vi "Module Info.vi"(8 "error in (no error)":errorcluster, 11 "BoardHandle":T2) -> (0 "error out":errorcluster, 2 "Module Info":T1, 3 "BoardHandle out":T2)   [LabVIEW 2020, in "CAEN PSM.lvlib"]
doc: "This function returns some information of the board."
uses:
  CAEN PSM.lvlib
  Private/BoardHandle.ctl
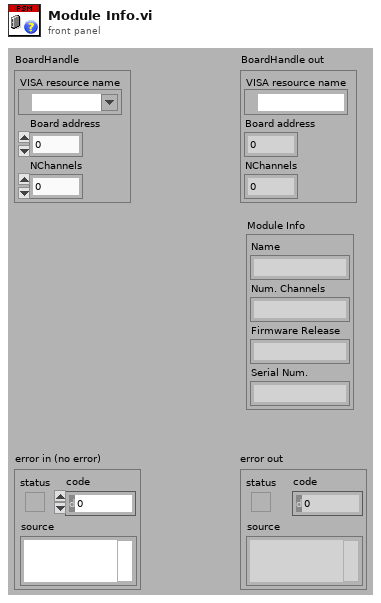
[diagram p1: front panel]
types:
  T1 = cluster{"Name":string, "Num. Channels":string, "Firmware Release":string, "Serial Num.":string}
  T2 = typedef "CAEN PSM.lvlib/BoardHandle.ctl" = cluster{"VISA resource name":refnum<visa-resource-name>, "Board address":i8, "NChannels":u8}
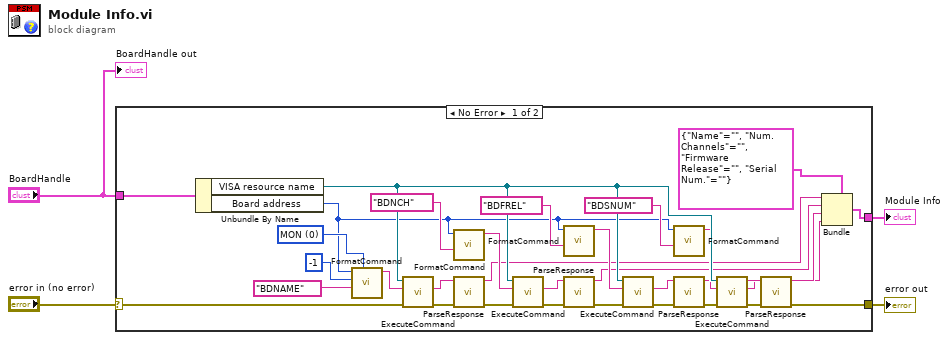
[diagram p0: block diagram]
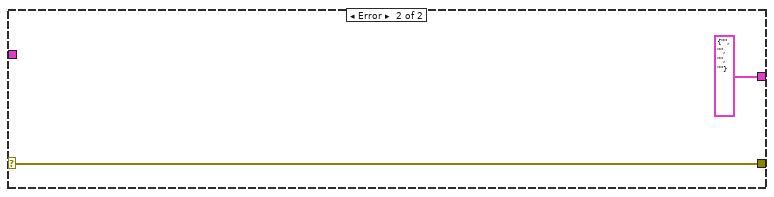
[diagram p2: hidden frame]
diagram:
  n1 = case shown="No Error" "error in (no error)" {
    selector: "error in (no error)" -> [w31 w38]
    tunnel: [w19 w38] -> w3
    tunnel: "BoardHandle" -> [w32 _]
    tunnel: [w9 T1 {"Name"="", "Num. Channels"="", "Firmware Release"="", "Serial Num."=""}] -> w1
    frame No Error {
      w36 = u8 0 items=["MON", "SET"] ("CMD")
      n2 = Unbundle By Name(w32) -> ("VISA resource name"=w18:refnum<visa-resource-name>, "Board address"=w8:i8)
      n3 = call "FormatCommand.vi"("CMD (MON)"=w36, "PAR"="BDNAME", "CH"=i8 -1, "BD (0)"=w8) -> ("cmd"=w35:string)  [unwired: 7 in]
      n4 = call "ExecuteCommand.vi"("error in (no error)"=w31, "Command"=w35, "VISA resource name"=w18) -> ("error out"=w34:errorcluster, "Response"=w33:string)  [unwired: 6 in, 1 out]
      n5 = call "FormatCommand.vi"("PAR"="BDNCH", "BD (0)"=w8) -> ("cmd"=w17:string)  [unwired: 9 in]
      n6 = call "ParseResponse.vi"("error in (no error)"=w34, "Response"=w33) -> ("error out"=w22:errorcluster, "val"=w13:string)  [unwired: 6 in, 2 out]
      n7 = call "ExecuteCommand.vi"("error in (no error)"=w22, "Command"=w17, "VISA resource name"=w18) -> ("error out"=w25:errorcluster, "Response"=w7:string)  [unwired: 6 in, 1 out]
      n8 = call "FormatCommand.vi"("PAR"="BDFREL", "BD (0)"=w8) -> ("cmd"=w16:string)  [unwired: 9 in]
      n9 = call "ParseResponse.vi"("error in (no error)"=w25, "Response"=w7) -> ("error out"=w21:errorcluster, "val"=w12:string)  [unwired: 6 in, 2 out]
      n10 = call "ExecuteCommand.vi"("error in (no error)"=w21, "Command"=w16, "VISA resource name"=w18) -> ("error out"=w24:errorcluster, "Response"=w6:string)  [unwired: 6 in, 1 out]
      n11 = call "FormatCommand.vi"("PAR"="BDSNUM", "BD (0)"=w8) -> ("cmd"=w15:string)  [unwired: 9 in]
      n12 = call "ParseResponse.vi"("error in (no error)"=w24, "Response"=w6) -> ("error out"=w20:errorcluster, "val"=w11:string)  [unwired: 6 in, 2 out]
      n13 = call "ExecuteCommand.vi"("error in (no error)"=w20, "Command"=w15, "VISA resource name"=w18) -> ("error out"=w23:errorcluster, "Response"=w5:string)  [unwired: 6 in, 1 out]
      n14 = call "ParseResponse.vi"("error in (no error)"=w23, "Response"=w5) -> ("error out"=w19:errorcluster, "val"=w10:string)  [unwired: 6 in, 2 out]
      n15 = Bundle(cluster=T1 {"Name"="", "Num. Channels"="", "Firmware Release"="", "Serial Num."=""}, "Name"=w13, "Num. Channels"=w12, "Firmware Release"=w11, "Serial Num."=w10) -> (w9:T1)
    }
    frame Error {
    }
  }
  "error out" <- w3
  "Module Info" <- w1
  "BoardHandle out" <- "BoardHandle"
